vi "Activation.vi"(8 "error in (no error)":errorcluster, 9 "Cell Position":T1, 10 "MenuRef":refnum<k9>, 11 "MCLB_Template in":refnum<class "MCLB_Template.lvclass">) -> (0 "error out":errorcluster, 3 "MCLB_Template out":refnum<class "MCLB_Template.lvclass">)   [LabVIEW 2021, in "MCLB_Template.lvclass"]
doc: "Shortcut Menu Activation?"
uses:
  MCLB_Template.lvclass
  MCLB_Template.lvclass/MCLB_Template.ctl
  <userlib>/John_Lib/Control_Lib/MCLB_Lib/MCLB_Lib.lvclass
  <vilib>/Utility/miscctls.llb/LVRowAndColumnTypeDef.ctl
panel:
  out "Array":string[](array[string])
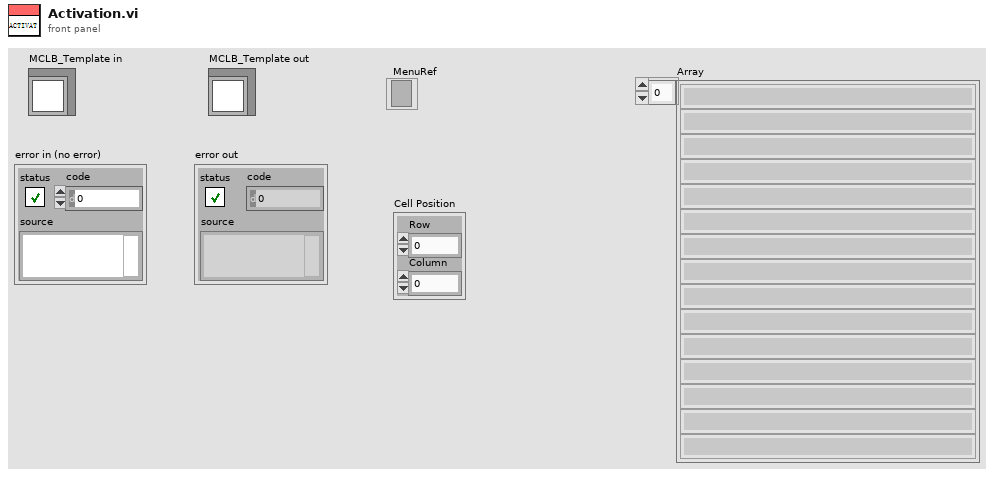
[diagram p1: front panel]
types:
  T1 = typedef "LVRowAndColumnTypeDef.ctl" = cluster{"Row":i32, "Column":i32}
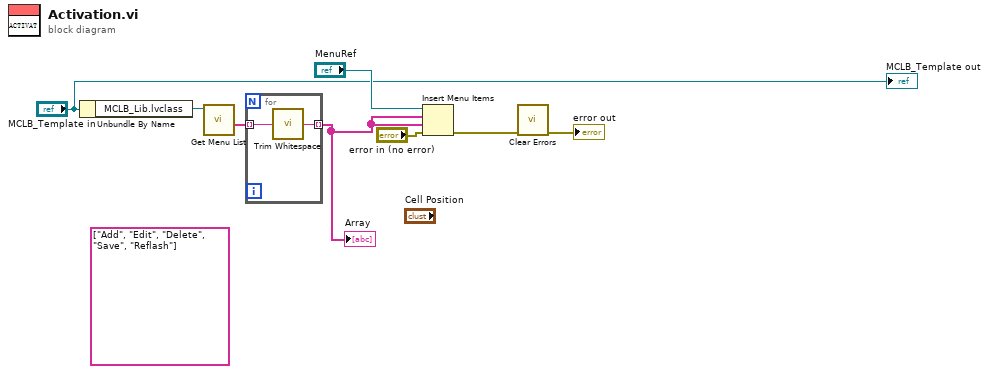
[diagram p0: block diagram]
diagram:
  (unwired) string[] ["Add", "Edit", "Delete", "Save", "Reflash"] ("Array")
  n1 = Unbundle By Name("MCLB_Template in") -> ("MCLB_Lib.lvclass"=w8:refnum<class "MCLB_Lib.lvclass">)
  n2 = call <userlib>:"Get Menu List.vi"("MCLB_Lib in"=w8) -> ("Menu En_Lis"=w4:string[])  [unwired: 7 in, 3 out]
  n3 = for {
    tunnel: w4 -> [w10] mode=indexing
    tunnel: [w9] -> w3 mode=indexing
    n4 = call <vilib>:"Trim Whitespace.vi"("string"=w10) -> ("trimmed string"=w9:string)  [unwired: 1 in]
  }
  "Array" <- w3
  n5 = Insert Menu Items(6:"error in (no error)", 7:w3, 8:w3, 9:"MenuRef") -> (0:w5:errorcluster)  [unwired: 2 in, 2 out]
  n6 = call <vilib>:"Clear Errors.vi"("error in (no error)"=w5) -> ("error out"=→"error out":errorcluster)  [unwired: 5 in, 1 out]
  "MCLB_Template out" <- "MCLB_Template in"
